vi "Read Label Props.vi"(8 "error in (no error)":errorcluster, 11 "Ctl Refnum in":refnum<vi>) -> (0 "error out":errorcluster, 2 "Label Props":T1, 3 "Ctl Refnum":refnum<vi>)   [LabVIEW 2020, in "VolatusGUIEditorCore.lvlib"]
uses:
  VolatusGUIEditorCore.lvlib
  Label Props.ctl
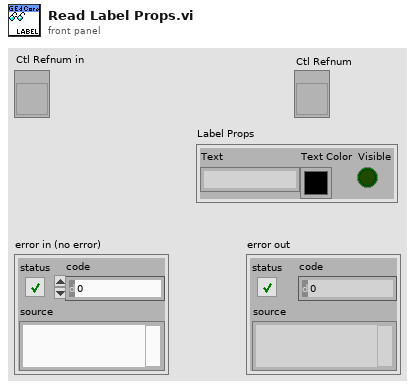
[diagram p1: front panel]
types:
  T1 = typedef "VolatusGUIEditorCore.lvlib/Label Props.ctl" = cluster{"Text":string, "Text Color":u32, "Visible":bool}
  T2 = cluster{"Label.Text":string, "Label.TextColor":u32, "Label.Visible":bool}
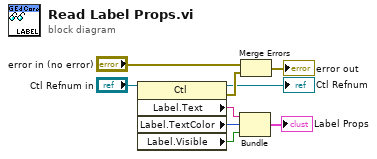
[diagram p0: block diagram]
diagram:
  n1 = property class="Ctl"(reference="Ctl Refnum in") -> (reference out=→"Ctl Refnum":refnum<vi>, error out=w7:errorcluster, "Label.Text"=w4:string, "Label.TextColor"=w3:u32, "Label.Visible"=w2:bool)  [unwired: 1 in]
  n2 = Bundle("Label.Text"=w4, "Label.TextColor"=w3, "Label.Visible"=w2) -> (→"Label Props":T2)  [unwired: 1 in]
  n3 = Merge Errors("error in (no error)", w7) -> (→"error out":errorcluster)
